vi "Plot Point (SubVI).vi"(8 "Polar Graph Attributes":T3, 9 "Array":T1(array[cluster]), 10 "grid measurements":T2, 11 "new picture in":picture) -> (3 "new picture":picture)   [LabVIEW 2020]
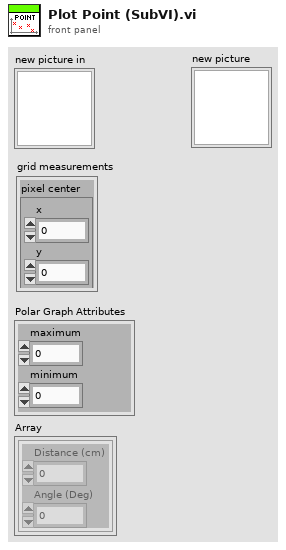
[diagram p1: front panel]
types:
  T1 = cluster{"Distance (cm)":dbl, "Angle (Deg)":dbl}[]
  T2 = cluster{"pixel center":cluster{"x":i16, "y":i16}, "scale factors":cluster{"a":dbl, "b":dbl, "log?":bool}, "grid color":u32, "start angle":dbl, "end angle":dbl, "tick length":i16, "pixel radius":i32}
  T3 = cluster{"maximum":dbl, "minimum":dbl, "clip to min":bool, "log?(F)":bool, "grid color":u32, "plot color":u32, "format and precision":cluster{"format":enum8{"Decimal", "Scientific", "Engineering", "Binary", "Octal", "Hex"}, "precision":u8}, "visible section":u16}
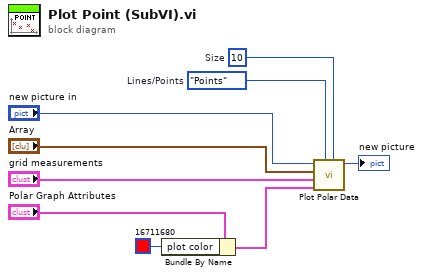
[diagram p0: block diagram]
diagram:
  w5 = u16 10  # Size
  w4 = enum16{"Lines", "Points"}."Points"  # Lines/Points
  n1 = Bundle By Name(cluster="Polar Graph Attributes", "plot color"=u32 16711680 ("Background Color")) -> (w9:T3)
  n2 = call <vilib>:"Plot Polar Data.vi"("Size"=w5, "Lines/Points"=w4, "polar attributes"=w9, "grid measurements"="grid measurements", "polar data"="Array", "picture"="new picture in") -> ("new picture"=→"new picture":picture)  [unwired: 3 in]
